vi "G#Object_Delete.vi"(0 "reference in":refnum<class "G#Object.lvclass">, 2 "force delete? (F)":bool, 5 "error in (no error)":errorcluster) -> (14 "reference out":refnum<class "G#Object.lvclass">, 19 "error out":errorcluster)   [LabVIEW 2020, in "G#Object.lvclass"]
doc: "Deletes the object if force delete is enabled, else it does nothing. The actual deleting of the object is done by the destructor, Destroy."
uses:
  G#Object.lvclass
  utils/G#Object_State.ctl
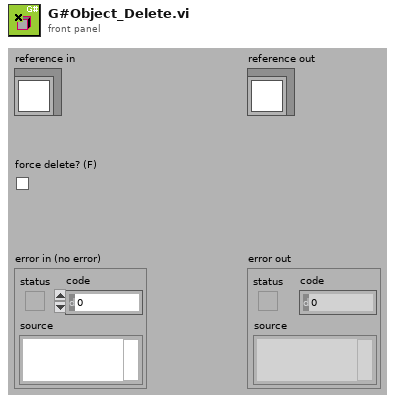
[diagram p1: front panel]
types:
  T1 = typedef "G#Object.lvclass/G#Object_State.ctl" = enum16{"Clear", "Create", "Delete", "Get class attributes", "Class hierarchy", "Get attribute value", "Set attribute value"}
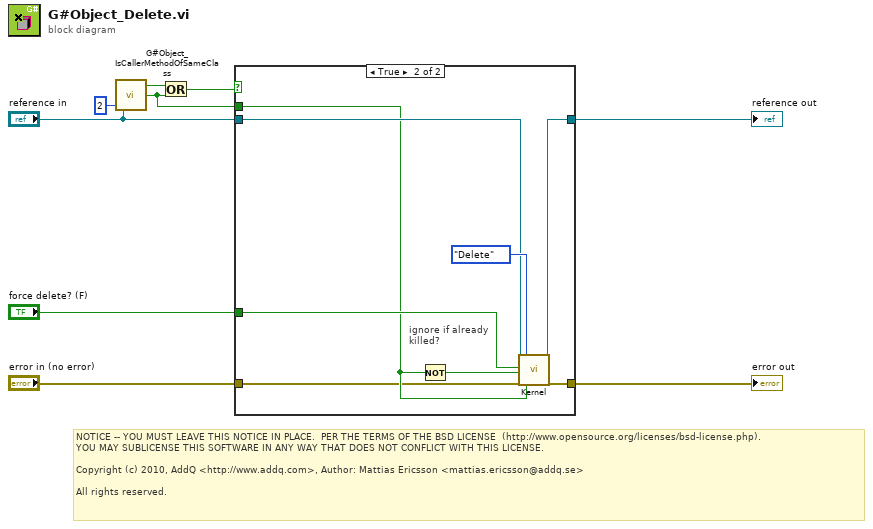
[diagram p0: block diagram]
diagram:
  # "NOTICE -- YOU MUST LEAVE THIS NOTICE IN PLACE.  PER THE TERMS OF THE BSD LICENSE  (http://www.opensource.org/licenses/bsd-license.php).\nYOU MAY SUBLICENSE THIS SOFTWARE IN ANY WAY THAT DOES NOT CONFLICT WITH THIS LICENSE.\n\nCopyright (c) 2010, AddQ <http://www.addq.com>, Author: Mattias Ericsson <mattias.ericsson@addq.se>\n\nAll rights reserved."
  n1 = call "G#Object_IsCallerMethodOfSameClass.vi"("call depth (1)"=2 ("call depth"), "reference in"="reference in") -> ("is caller of G#Object?"=w1:bool, "is of same class?"=w3:bool)  [unwired: 1 in, 1 out]
  n2 = Or(x=w3, y=w1) -> (x .or. y?=w2:bool)
  n3 = case shown="True" w2 {
    tunnel: [w11 w19] -> w9
    tunnel: "error in (no error)" -> [w11 w12]
    tunnel: "force delete? (F)" -> [_ w15]
    tunnel: "reference in" -> [w10 w16]
    tunnel: [w10 w17] -> w4
    tunnel: w1 -> [_ w13]
    frame False {
    }
    frame True {
      # "ignore if already\nkilled?"
      n4 = Not(x=w13) -> (.not. x?=w14:bool)
      n5 = call-dynamic "Kernel.vi"("reference in"=w16, "option 1"=w15, "option 2"=w14, "error in (no error)"=w12, "state"=G#Object_State."Delete" ("State"), "option 3"=w13) -> ("reference out"=w17:refnum<class "G#Object.lvclass">, "error out"=w19:errorcluster)  [unwired: 5 in, 7 out]
    }
  }
  "error out" <- w9
  "reference out" <- w4
